vi "Popup Launcher.vi"(6 "Panel":refnum<class "Panel.lvclass">, 8 "error in (no error)":errorcluster, 9 "Popup Return Data":refnum<user-event>, 10 "String in":string, 11 "Generic Data Type in":refnum<class "Generic Data Type.lvclass">) -> (0 "error out":errorcluster, 3 "Generic Data Type out":refnum<class "Generic Data Type.lvclass">)   [LabVIEW 2018, in "Generic Data Type.lvclass"]
uses:
  Generic Data Type.lvclass
  <vilib>/MGI/Panel Manager/Panel/Panel/Panel.lvclass
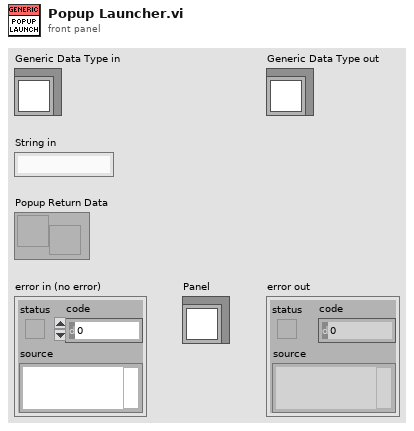
[diagram p1: front panel]
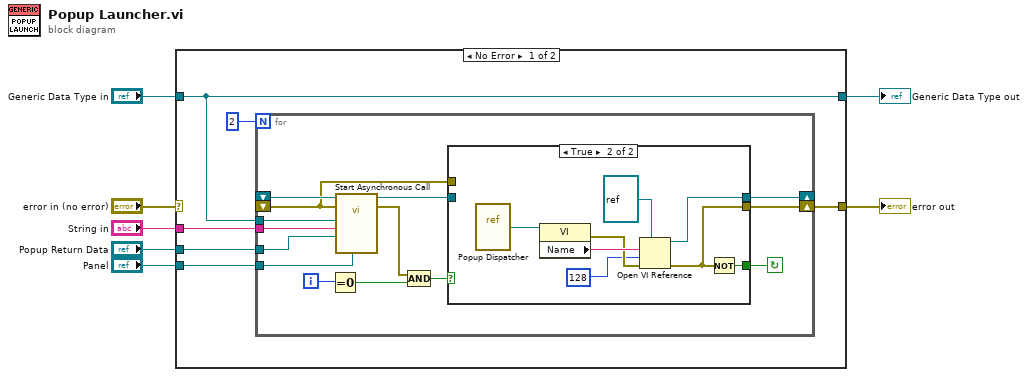
[diagram p0: block diagram]
diagram:
  n1 = case shown="No Error" "error in (no error)" {
    selector: "error in (no error)" -> [_ w39]
    tunnel: [w11 w39] -> w6
    tunnel: [w12 w38] -> w4
    tunnel: "Generic Data Type in" -> [w12 w38]
    tunnel: "String in" -> [w10 _]
    tunnel: "Popup Return Data" -> [w9 _]
    tunnel: "Panel" -> [w8 _]
    frame No Error {
      n2 = for {
        N: 2 -> [_]
        tunnel: w12 -> [w27]
        shift-right: [w24] -> _
        shift-left: _ -> [w26]
        shift-right: [w18] -> w11
        shift-left: _ -> [w17]
        tunnel: w10 -> [w16]
        tunnel: w9 -> [w15]
        tunnel: w8 -> [w14]
        i -> [w22]
        stop <- w23 continue-if-true
        n3 = Equal To 0?(x=w22) -> (x = 0?=w21:bool)
        n4 = call-by-ref "Start Asynchronous Call"(reference=w26, error in=w17, "Panel"=w14, "Popup Return Data"=w15, "String in"=w16, "Generic Data Type in"=w27) -> (reference out=w25:refnum<vi>, error out=w20:errorcluster)  [unwired: 6 in, 2 out]
        n5 = Compound Arithmetic op=AND(w20, w21) -> (w19:bool)
        n6 = case shown="True" w19 {
          tunnel: w25 -> [w29 _]
          tunnel: [w29 w32] -> w24
          tunnel: [_ w31] -> w23
          tunnel: [w28 w30] -> w18
          tunnel: w17 -> [w28 _]
          frame False {
          }
          frame True {
            n7 = vi-ref "Popup Dispatcher.vi"() -> (w37:refnum<vi>)
            n8 = property class="VI"(reference=w37) -> (error out=w35:errorcluster, "Name"=w36:string)  [unwired: 1 in, 1 out]
            n9 = Open VI Reference(type specifier VI Refnum (for type only)=refnum<vi> refnum, vi path=w36, options=128, error in (no error)=w35) -> (vi reference=w32:refnum<vi>, error out=w30:errorcluster)  [unwired: 2 in]
            n10 = Not(x=w30) -> (.not. x?=w31:bool)
          }
        }
      }
    }
    frame Error {
    }
  }
  "error out" <- w6
  "Generic Data Type out" <- w4
